vi "test.vi"   [LabVIEW 2014]
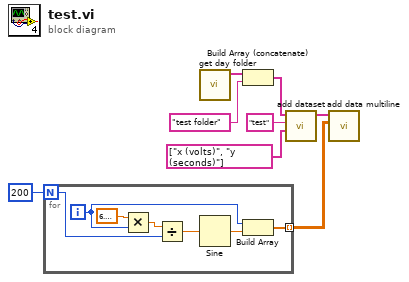
[diagram p0: block diagram]
diagram:
  n1 = for {
    N: 200 -> [w14]
    tunnel: [w9] -> w2 mode=indexing
    i -> [w11]
    n2 = Multiply(x=6.283185307179586, y=w11) -> (x*y=w13:dbl)
    n3 = Divide(x=w13, y=w14) -> (x/y=w12:dbl)
    n4 = Sine(x=w12) -> (sin(x)=w10:dbl)
    n5 = Build Array(w11, w10) -> (w9:dbl[])
  }
  n6 = call "get day folder.vi"() -> ("day folder"=w7:string[])  [unwired: 10 in, 1 out]
  n7 = Build Array (concatenate)(w7, "test folder" ("name")) -> (w5:string[])
  n8 = call "add dataset.vi"("fields"=string[] ["x (volts)", "y (seconds)"], "name"="test", "folder"=w5) -> ("path"=w1:string[])  [unwired: 7 in, 1 out]
  n9 = call "add data multiline.vi"("data"=w2, "path"=w1) -> ()  [unwired: 9 in, 1 out]
